vi "Query.vi"(0 "reference in":refnum<class "Database_Postgress.lvclass">, 5 "Query":string, 7 "Timeout":i32=10000, 11 "error in (no error)":errorcluster) -> (4 "reference out":refnum<class "Database_Postgress.lvclass">, 6 "Query Return":T1[](array[typedef]), 15 "error out":errorcluster)   [LabVIEW 2019, in "Database_Postgress.lvclass"]
uses:
  Database_Postgress.lvclass
  Query Return.ctl
  Database_Postgress.lvclass/Database_Postgress.ctl
  Neosoft Technologies/NeoDB for PostgreSQL/Postgres Connector/Postgres Connector.lvclass
  DatabaseInterface_class/DatabaseInterface.lvclass
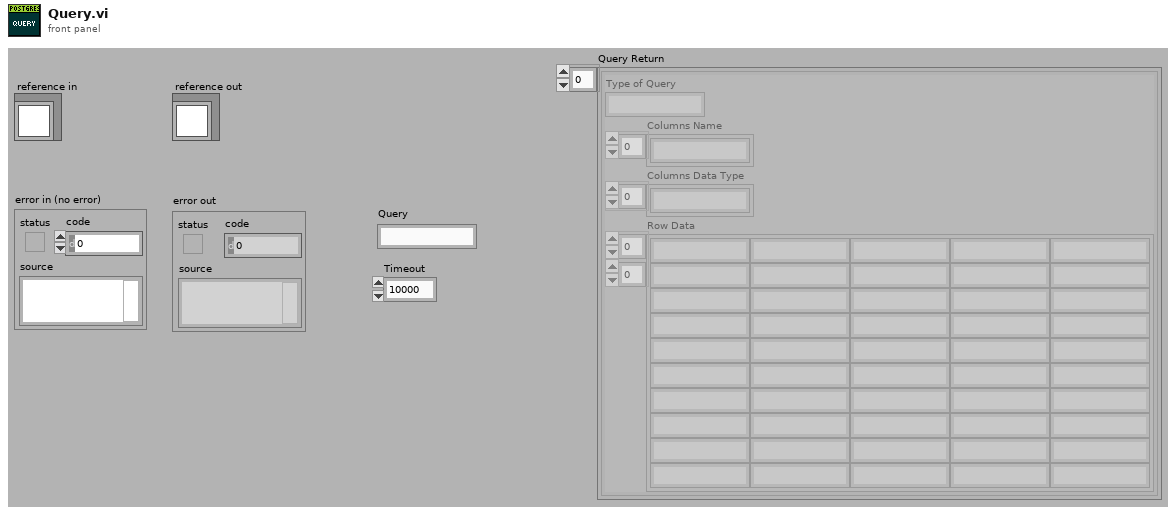
[diagram p1: front panel]
types:
  T1 = typedef "DatabaseInterface.lvclass/Query Return.ctl" = cluster{"Type of Query":string, "Columns Name":string[], "Columns Data Type":string[], "Row Data":string[][]}
  T2 = typedef "PG_LIB.lvlib/Postgres Connector.lvclass/Cluster_Return_Of_The_Query.ctl" = cluster{"Type of Query":string, "Columns Name":string[], "Columns Data Type":string[], "Row Data":string[][]}
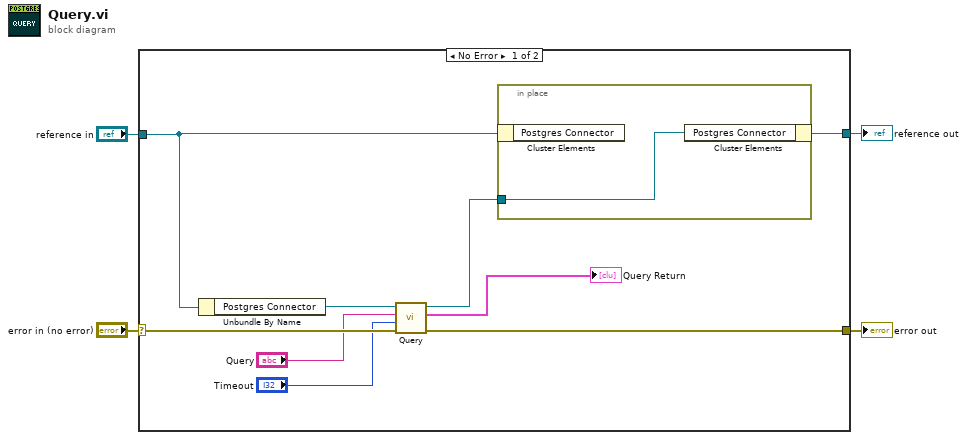
[diagram p0: block diagram]
diagram:
  n1 = case shown="No Error" "error in (no error)" {
    selector: "error in (no error)" -> [w13 w16]
    tunnel: [w9 w16] -> w1
    tunnel: [w5 w15] -> w2
    tunnel: "reference in" -> [w12 w15]
    frame No Error {
      n2 = Unbundle By Name(w12) -> ("Postgres Connector"=w10:refnum<class "Postgres Connector.lvclass">)
      n3 = call "Query.vi"("error in (no error)"=w13, "Timeout"="Timeout", "Query"="Query", "Postgres Connector In"=w10) -> ("error out"=w9:errorcluster, "Query Return"=→"Query Return":T2[], "Postgres Connector Out"=w11:refnum<class "Postgres Connector.lvclass">)  [unwired: 5 in]
      n4 = in-place {
        in-place-border: w11 -> [w14]
        n5 = in-place-cluster #1(w12) -> ()  [unwired: 1 out]
        n6 = in-place-cluster #1("Postgres Connector"=w14) -> (w5:refnum<class "Database_Postgress.lvclass">)
      }
    }
    frame Error {
    }
  }
  "error out" <- w1
  "reference out" <- w2
